vi "cc_write.vi"(3 "error in (no error)":errorcluster, 4 "Output Command":string, 5 "VISA In":refnum<visa-resource-name>) -> (0 "error out":errorcluster, 2 "VISA Out":refnum<visa-resource-name>)   [LabVIEW 2020]
doc: "Write a string command to Cryocon."
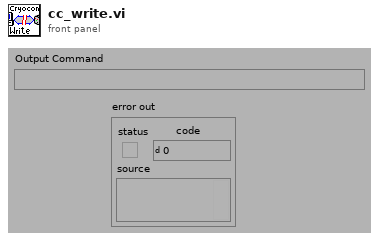
[diagram p1: front panel]
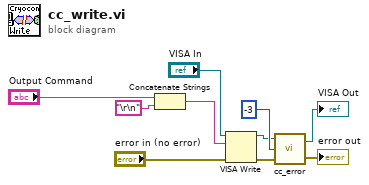
[diagram p0: block diagram]
diagram:
  n1 = Concatenate Strings("Output Command", "\r\n") -> (w1:string)
  n2 = VISA Write(VISA resource name="VISA In", write buffer=w1, error in (no error)="error in (no error)") -> (VISA resource name out=w5:refnum<visa-resource-name>, error out=w7:errorcluster)  [unwired: 1 out]
  n3 = call "cc_error.vi"("error in (no error)"=w7, "Error code"=-3, "VISA In"=w5) -> ("error out"=→"error out":errorcluster, "VISA out"=→"VISA Out":refnum<visa-resource-name>)
